vi "init.vi"(8 "error in (no error)":errorcluster, 11 "Protocol_B in":refnum<class "Protocol_B.lvclass">) -> (0 "error out":errorcluster, 3 "Protocol_B out":refnum<class "Protocol_B.lvclass">)   [LabVIEW 2011, in "Protocol_B.lvclass"]
uses:
  Protocol_B.lvclass
  protocol_Generic/Protocol_Generic.lvclass
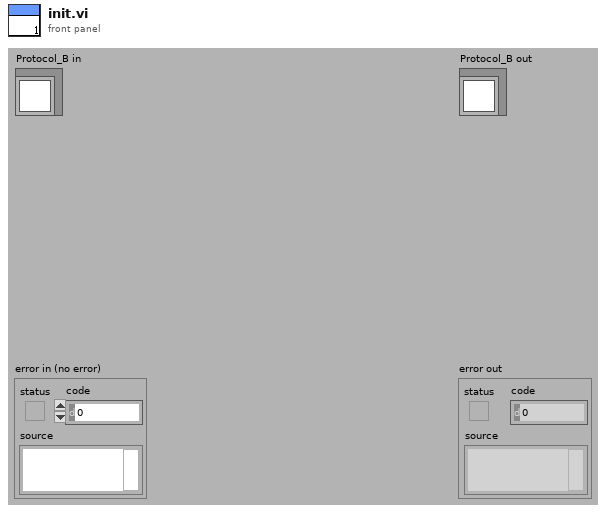
[diagram p1: front panel]
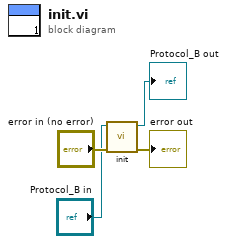
[diagram p0: block diagram]
diagram:
  n1 = call-parent "init.vi"("error in (no error)"="error in (no error)", "Protocol_Generic in"="Protocol_B in") -> ("error out"=→"error out":errorcluster, "Protocol_Generic out"=→"Protocol_B out":refnum<class "Protocol_B.lvclass">)  [unwired: 8 in]
